vi "sound_ctrl.vi"(8 "Volume":fxp<+,64,32>, 9 "frequency (periods/tick)":fxp<+,32,0>, 11 "stop":bool) -> (1 "AccelerationZ":i16, 2 "AccelerationY":i16, 3 "AccelerationX":i16)   [LabVIEW 2016]
uses:
  <vilib>/rvi/Emulation/niFpgaGetClockAttributes.vi
  <vilib>/rvi/Emulation/niFpgaSctlEmulationGetInTimedLoop.vi
  <vilib>/rvi/Emulation/niFpgaEmulationReportErrorSimple.vi
  <vilib>/rvi/eio/common/nirviEmuTemplateMethod_errors.vi
  <vilib>/rvi/Emulation/niFpgaCriticalErrorInLSC.vi
  <vilib>/rvi/FXPMathLib/FxpAdd/XNode/nifxpmath_Add.xnode
  <vilib>/eio/EIONode/EIONode.xnode
  <vilib>/rvi/FXPMathLib/sim/FxpSim.dll
panel:
  in  "frequency (periods/tick) 2":fxp<+,32,0>
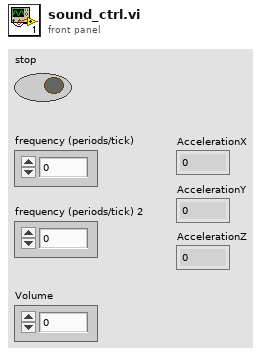
[diagram p1: front panel]
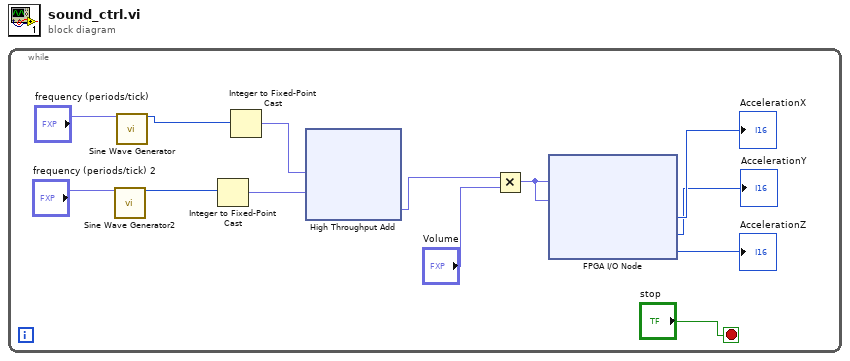
[diagram p0: block diagram]
diagram:
  n1 = while {
    stop <- "stop" stop-if-true
    n2 = call "Sine Wave Generator2"("frequency (periods/tick)"="frequency (periods/tick) 2") -> ("sine out"=w3:i16)  [unwired: 14 in]
    n3 = call "Sine Wave Generator"("frequency (periods/tick)"="frequency (periods/tick)") -> ("sine out"=w5:i16)  [unwired: 14 in]
    n4 = Integer to Fixed-Point Cast(integer=w3) -> (fixed-point=w2:fxp<+/-,16,16>)  [unwired: 1 in]
    n5 = Integer to Fixed-Point Cast(integer=w5) -> (fixed-point=w4:fxp<+/-,16,16>)  [unwired: 1 in]
    n6 = xnode "High Throughput Add"("x"=w4, "y"=w2) -> ("x+y"=w1:fxp<+/-,17,17>)
    n7 = Multiply(x=w1, y="Volume") -> (x*y=w11:fxp<+/-,64,49>)
    n8 = xnode "FPGA I/O Node"("AudioOut/Left"=w11, "AudioOut/Right"=w11) -> ("AccelerationX"=→"AccelerationX":i16, "AccelerationY"=→"AccelerationY":i16, "AccelerationZ"=→"AccelerationZ":i16)  [unwired: 5 in, 5 out]
  }
